vi "Lock Mutex.vi"(8 "error in (no error)":errorcluster, 10 "Owner":string, 11 "Mutex In":T1) -> (0 "error out":errorcluster, 3 "Mutex Out":T1)   [LabVIEW 2021]
uses:
  <vilib>/myRIO/Common/Instrument Driver Framework/Utilities/typedefs/Reentrant Mutex.ctl
panel:
  in  "Reentrant?":bool
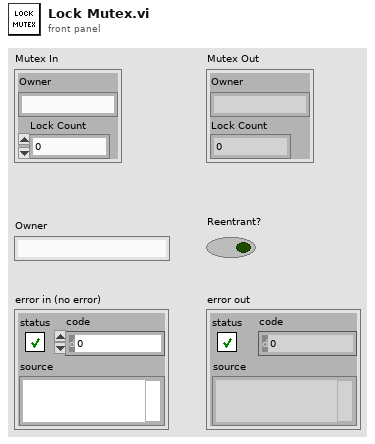
[diagram p1: front panel]
types:
  T1 = typedef "Reentrant Mutex.ctl" = cluster{"Owner":string, "Lock Count":u32}
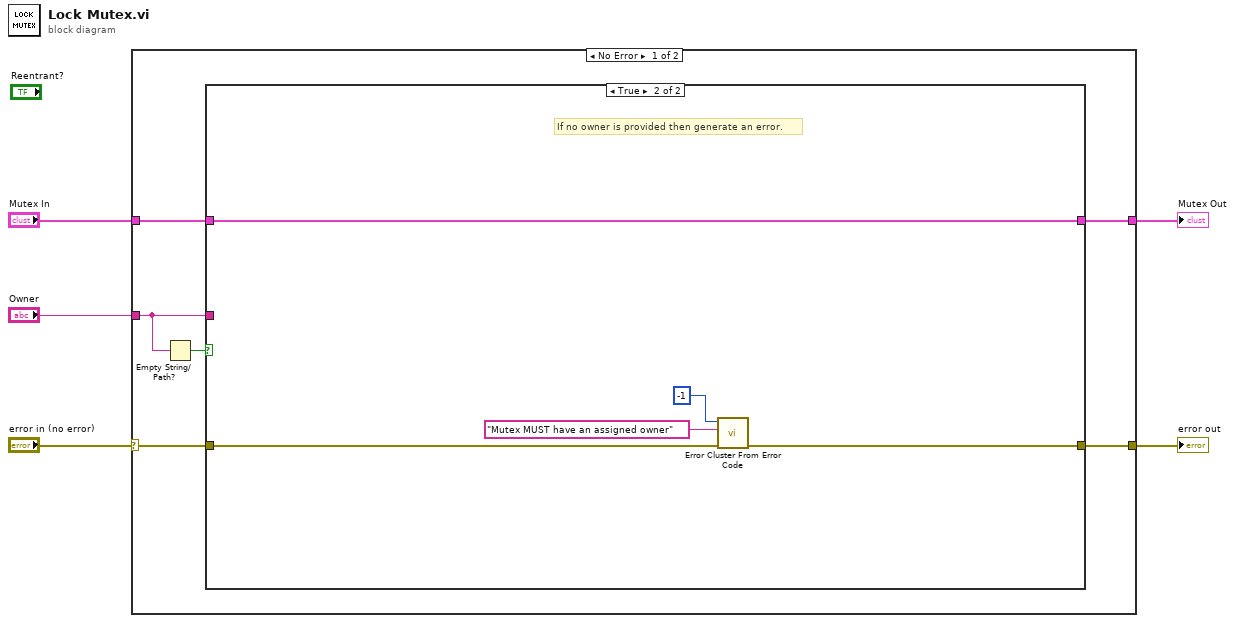
[diagram p0: block diagram]
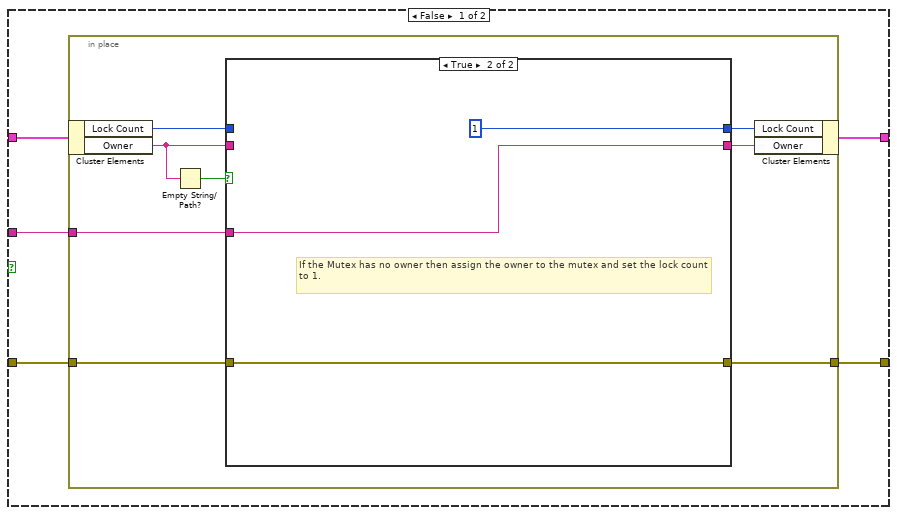
[diagram p2: hidden frame]
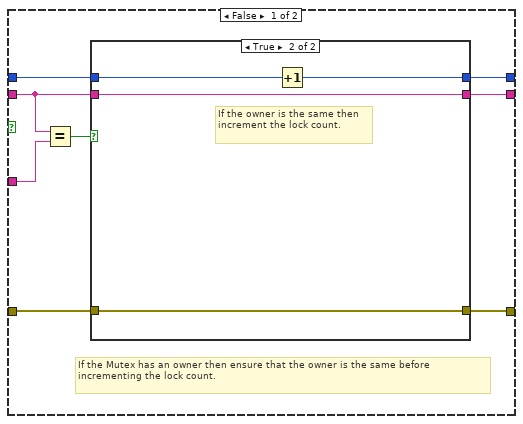
[diagram p3: hidden frame]
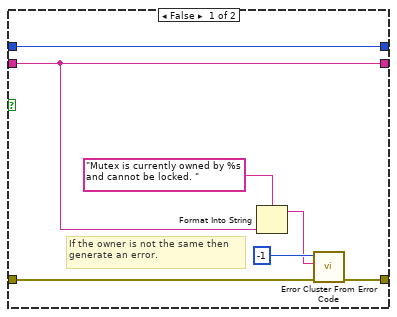
[diagram p4: hidden frame]
diagram:
  n1 = case shown="No Error" "error in (no error)" {
    selector: "error in (no error)" -> [w10 w53]
    tunnel: "Mutex In" -> [w8 w52]
    tunnel: "Owner" -> [w6 _]
    tunnel: [w9 w53] -> w2
    tunnel: [w7 w52] -> w1
    frame No Error {
      n2 = Empty String/Path?(string/path=w6) -> (empty?=w11:bool)
      n3 = case shown="True" w11 {
        tunnel: w10 -> [w16 w51]
        tunnel: [w14 w50] -> w9
        tunnel: w8 -> [w13 w47]
        tunnel: w6 -> [w15 _]
        tunnel: [w12 w47] -> w7
        frame False {
          n4 = in-place {
            in-place-border: w16 -> [w24]
            in-place-border: w15 -> [w23]
            in-place-border: [w21] -> w14
            n5 = in-place-cluster #1(w13) -> ("Lock Count"=w20:u32, "Owner"=w17:string)
            n6 = Empty String/Path?(string/path=w17) -> (empty?=w22:bool)
            n7 = case shown="True" w22 {
              tunnel: w24 -> [w26 w46]
              tunnel: w23 -> [w32 w45]
              tunnel: [w28 w45] -> w18
              tunnel: [w25 w46] -> w21
              tunnel: [w29 u32 1 ("Lock Count")] -> w19
              tunnel: w20 -> [w30 _]
              tunnel: w17 -> [w27 _]
              frame False {
                # "If the Mutex has an owner then ensure that the owner is the same before incrementing the lock count."
                n8 = Equal?(x=w27, y=w32) -> (x = y?=w31:bool)
                n9 = case shown="True" w31 {
                  tunnel: w30 -> [w39 w43]
                  tunnel: [w39 w42] -> w29
                  tunnel: [w34 w41] -> w28
                  tunnel: w27 -> [w34 w41]
                  tunnel: w26 -> [w37 w40]
                  tunnel: [w36 w40] -> w25
                  frame False {
                    # "If the owner is not the same then generate an error."
                    n10 = Format Into String(format string="Mutex is currently owned by %s  and cannot be locked. " ("error message (\"\")"), w34) -> (resulting string=w33:string)  [unwired: 2 in, 1 out]
                    n11 = call <vilib>:"Error Cluster From Error Code.vi"("error in (no error)"=w37, "error message (\"\")"=w33, "error code (0)"=-1) -> ("error out"=w36:errorcluster)  [unwired: 6 in]
                  }
                  frame True {
                    # "If the owner is the same then increment the lock count."
                    n12 = Increment(x=w43) -> (x+1=w42:u32)
                  }
                }
              }
              frame True {
                # "If the Mutex has no owner then assign the owner to the mutex and set the lock count to 1."
              }
            }
            n13 = in-place-cluster #1("Lock Count"=w19, "Owner"=w18) -> (w12:T1)
          }
        }
        frame True {
          # "If no owner is provided then generate an error."
          n14 = call <vilib>:"Error Cluster From Error Code.vi"("error in (no error)"=w51, "error message (\"\")"="Mutex MUST have an assigned owner" ("error message (\"\")"), "error code (0)"=-1) -> ("error out"=w50:errorcluster)  [unwired: 6 in]
        }
      }
    }
    frame Error {
    }
  }
  "Mutex Out" <- w1
  "error out" <- w2
